vi "SHORTED.vi"(10 "Input Data":dbl[](array[numeric]), 11 "Mean In":dbl=1600.0) -> (3 "SHORTED":bool)   [LabVIEW 2012]
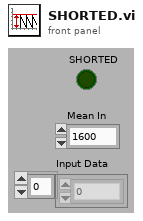
[diagram p1: front panel]
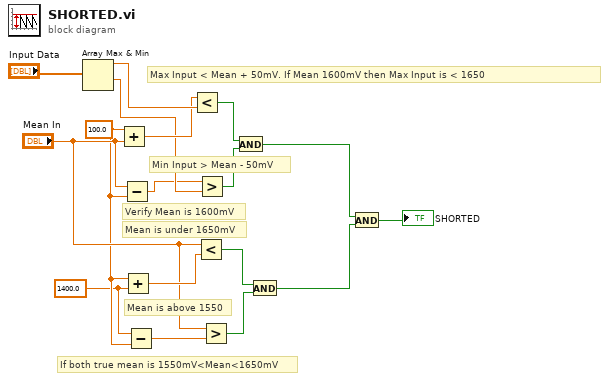
[diagram p0: block diagram]
diagram:
  w12 = 1400.0
  w13 = 100.0
  # "Min Input > Mean - 50mV"
  # "Max Input < Mean + 50mV. If Mean 1600mV then Max Input is < 1650"
  # "If both true mean is 1550mV<Mean<1650mV"
  # "Mean is above 1550"
  # "Mean is under 1650mV"
  # "Verify Mean is 1600mV"
  n1 = Array Max & Min(array="Input Data") -> (max value=w4:dbl, min value=w2:dbl)  [unwired: 2 out]
  n2 = Add(x=w13, y="Mean In") -> (x+y=w3:dbl)
  n3 = Subtract(x="Mean In", y=w13) -> (x-y=w1:dbl)
  n4 = Add(x=w13, y=w12) -> (x+y=w16:dbl)
  n5 = Subtract(x=w12, y=w13) -> (x-y=w15:dbl)
  n6 = Less?(x=w3, y=w4) -> (x < y?=w11:bool)
  n7 = Less?(x="Mean In", y=w16) -> (x < y?=w9:bool)
  n8 = Greater?(x=w1, y=w2) -> (0:w10:bool)
  n9 = Greater?(x="Mean In", y=w15) -> (0:w8:bool)
  n10 = And(x=w11, y=w10) -> (x .and. y?=w7:bool)
  n11 = And(x=w9, y=w8) -> (x .and. y?=w6:bool)
  n12 = And(x=w7, y=w6) -> (x .and. y?=→"SHORTED":bool)
